vi "Configure Precision Probe.vi"(0 "VISA resource name":refnum<visa-resource-name>, 1 "Precision Type (0: Probe)":i32(ring) items=["Probe", "Cable"], 2 "Bandwidth Limit (3)":dbl=3.0, 5 "Channel (1: Channel 1)":i32(ring)=1 items=["Channel 1"=1, "Channel 2"=2, "Channel 3"=3, "Channel 4"=4], 7 "Limit Type (0: Auto)":i32(ring) items=["Auto", "MAN", "BOOS"], 9 "Calibration Name (\"2-8-2\")":string="2-8-2", 11 "error in (no error)":errorcluster, 12 "Vtype (0: Vout/Vin)":i32(ring) items=["Vout/Vin", "Vout/Vsource"], 13 "Vsource Value ()":string) -> (4 "VISA resource name out":refnum<visa-resource-name>, 15 "error out":errorcluster)   [LabVIEW 2020, in "Agilent 90000 Series.lvlib"]
doc: "Configures settings for the PrecisionProbe or PrecisionCable."
uses:
  Agilent 90000 Series.lvlib
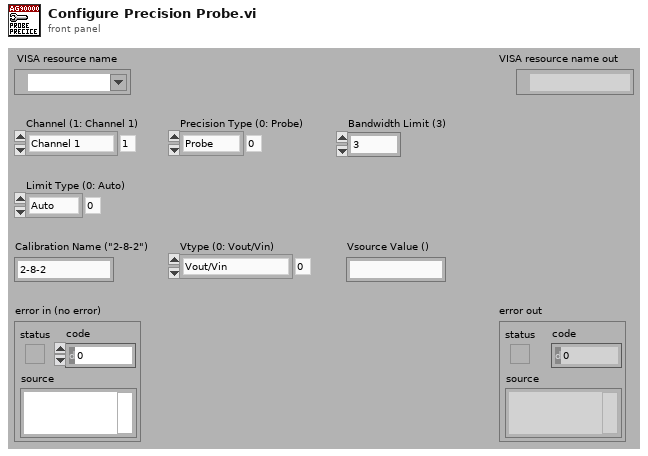
[diagram p1: front panel]
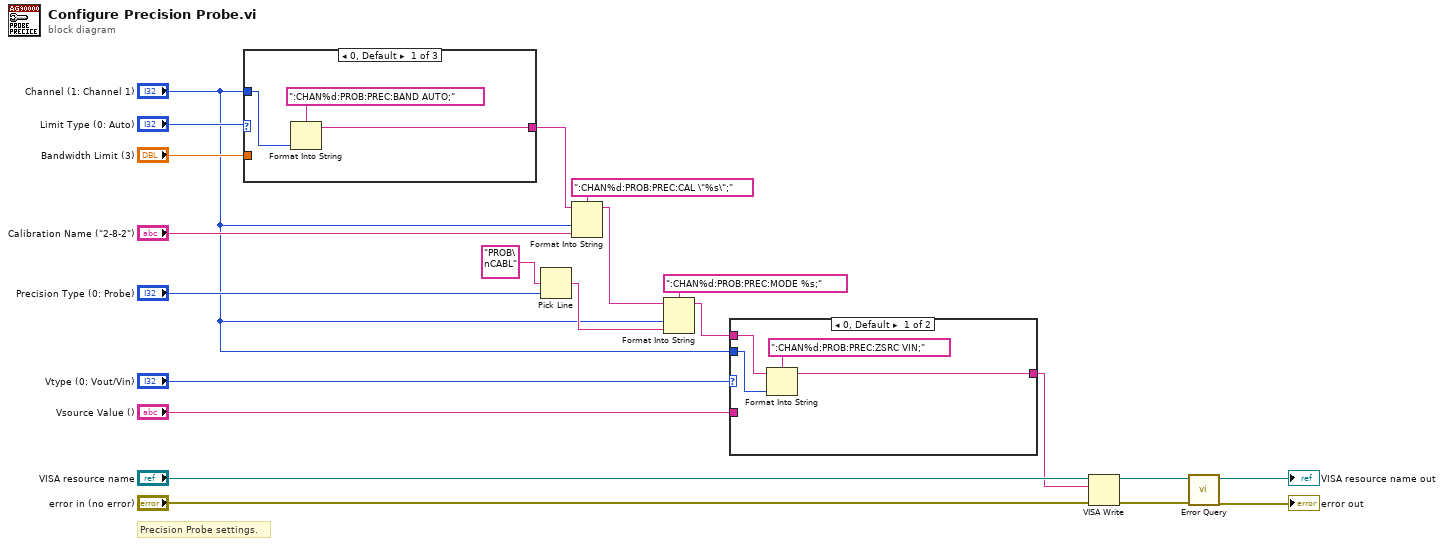
[diagram p0: block diagram]
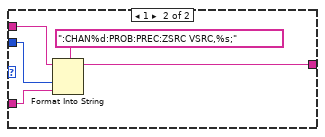
[diagram p2: hidden frame]
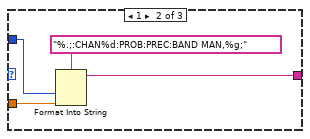
[diagram p3: hidden frame]
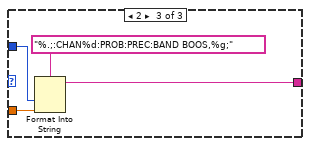
[diagram p4: hidden frame]
diagram:
  # "Precision Probe settings."
  n1 = case shown="0, Default" "Limit Type (0: Auto)" {
    tunnel: "Channel (1: Channel 1)" -> [w23 w27 w31]
    tunnel: "Bandwidth Limit (3)" -> [_ w26 w29]
    tunnel: [w22 w25 w30] -> w6
    frame 0, Default {
      n2 = Format Into String(format string=":CHAN%d:PROB:PREC:BAND AUTO;", w23) -> (resulting string=w22:string)  [unwired: 2 in, 1 out]
    }
    frame 1 {
      n3 = Format Into String(format string="%.;:CHAN%d:PROB:PREC:BAND MAN,%g;", w27, w26) -> (resulting string=w25:string)  [unwired: 2 in, 1 out]
    }
    frame 2 {
      n4 = Format Into String(format string="%.;:CHAN%d:PROB:PREC:BAND BOOS,%g;", w31, w29) -> (resulting string=w30:string)  [unwired: 2 in, 1 out]
    }
  }
  n5 = Pick Line(multi-line string="PROB\nCABL", line index="Precision Type (0: Probe)") -> (output string=w15:string)  [unwired: 1 out]
  n6 = Format Into String(format string=":CHAN%d:PROB:PREC:CAL \"%s\";", initial string=w6, "Channel (1: Channel 1)", "Calibration Name (\"2-8-2\")") -> (resulting string=w17:string)  [unwired: 1 in, 1 out]
  n7 = Format Into String(format string=":CHAN%d:PROB:PREC:MODE %s;", initial string=w17, "Channel (1: Channel 1)", w15) -> (resulting string=w2:string)  [unwired: 1 in, 1 out]
  n8 = case shown="0, Default" "Vtype (0: Vout/Vin)" {
    tunnel: "Channel (1: Channel 1)" -> [w36 w40]
    tunnel: "Vsource Value ()" -> [_ w39]
    tunnel: [w34 w37] -> w1
    tunnel: w2 -> [w33 w38]
    frame 0, Default {
      n9 = Format Into String(format string=":CHAN%d:PROB:PREC:ZSRC VIN;", initial string=w33, w36) -> (resulting string=w34:string)  [unwired: 1 in, 1 out]
    }
    frame 1 {
      n10 = Format Into String(format string=":CHAN%d:PROB:PREC:ZSRC VSRC,%s;", initial string=w38, w40, w39) -> (resulting string=w37:string)  [unwired: 1 in, 1 out]
    }
  }
  n11 = VISA Write(VISA resource name="VISA resource name", write buffer=w1, error in (no error)="error in (no error)") -> (VISA resource name out=w12:refnum<visa-resource-name>, error out=w11:errorcluster)  [unwired: 1 out]
  n12 = call "Error Query.vi"("error in (no error)"=w11, "VISA resource name"=w12) -> ("error out"=→"error out":errorcluster, "VISA resource name out"=→"VISA resource name out":refnum<visa-resource-name>)  [unwired: 8 out]
